vi "主UI.vi"() -> ()   [LabVIEW 2016, in "数据传输系统-03.lvlib" / "自动更新.lvlib" / "TCP文件传输系统.lvlib"]
uses:
  <vilib>/Utility/sysdir.llb/System Directory Type.ctl
panel:
  out "TCP接收全局簇":T1
  out "传输次数":dbl
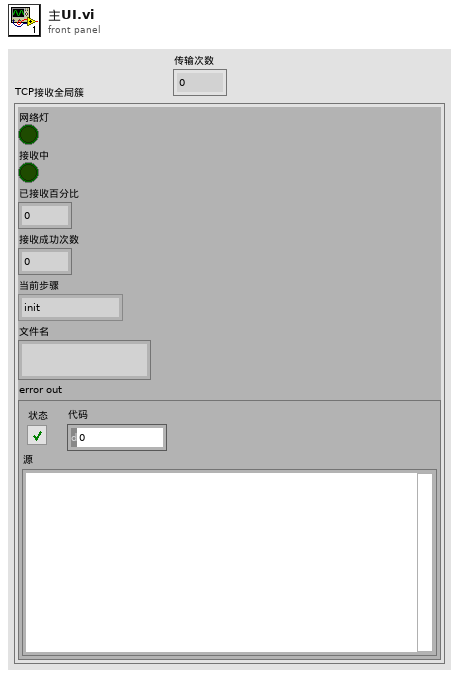
[diagram p1: front panel]
types:
  T1 = cluster{"网络灯":bool, "接收中":bool, "已接收百分比":u8, "接收成功次数":dbl, "当前步骤":enum16{"init", "receivehead", "receivecontent", "receivesuccess", "over"}, "文件名":string, "error out":errorcluster}
  T2 = typedef "System Directory Type.ctl" = i32
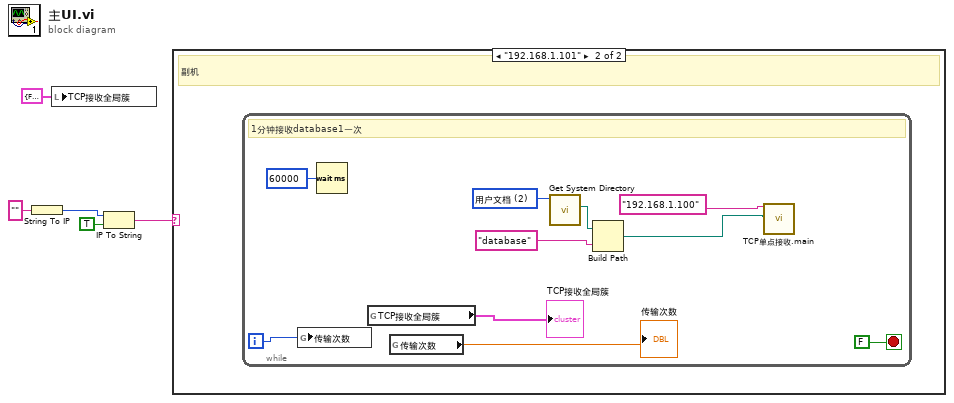
[diagram p0: block diagram]
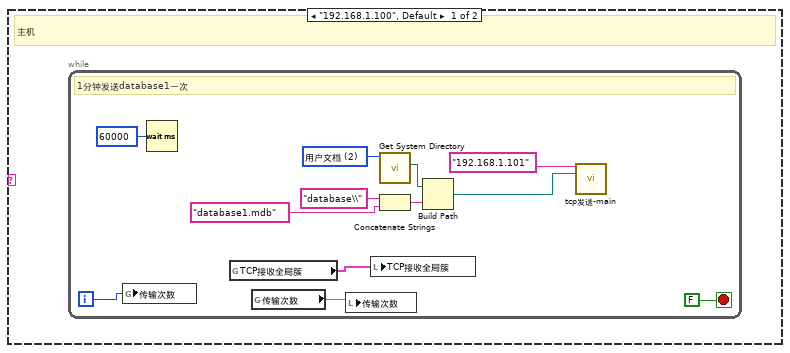
[diagram p2: hidden frame]
diagram:
  n1 = String To IP(1:"" ("名称")) -> (0:w5:u32)
  n2 = local write "TCP接收全局簇"(T1 {"网络灯"=FALSE, "接收中"=FALSE, "已接收百分比"=0, "接收成功次数"=0.0, "当前步骤"=enum."init", "文件名"="", "error out"={"status"=FALSE, "code"=0, "source"=""}} ("TCP接收全局簇")) -> ()
  n3 = IP To String(1:TRUE ("句点符号？(F)"), 2:w5) -> (0:w2:string)
  n4 = case shown="\"192.168.1.101\"" w2 {
    frame "192.168.1.100", Default {
      # "主机"
      n5 = while {
        i -> [w8]
        stop <- FALSE stop-if-true
        w14 = T2 2 items=["用户目录"=0, "用户桌面"=1, "用户文档"=2, "用户应用程序数据"=3, "用户设置"=4, "用户临时目录"=5, "公共文档"=6, "公共应用程序数据"=7, "公共设置"=8, "公共缓存"=13, "系统核心库"=9, "系统安装库"=10, "应用程序文件"=11, "启动盘根目录"=12] ("system directory type")
        # "1分钟发送database1一次"
        n6 = global write "全局变量1.vi" "传输次数"(w8) -> ()
        n7 = Wait (ms)(milliseconds to wait=u32 60000 ("等待时间（毫秒）")) -> ()  [unwired: 1 out]
        n8 = global read "全局变量1.vi" "TCP接收全局簇"() -> (w6:T1)
        n9 = global read "全局变量1.vi" "传输次数"() -> (w7:dbl)
        n10 = local write "传输次数"(w7) -> ()
        n11 = local write "TCP接收全局簇"(w6) -> ()
        n12 = call <vilib>:"Get System Directory.vi"("system directory type"=w14) -> ("system directory"=w13:path)  [unwired: 10 in]
        n13 = Concatenate Strings("database\\" ("condition"), "database1.mdb" ("字符串")) -> (w11:string)
        n14 = Build Path(base path=w13, name or relative path=w11) -> (appended path=w9:path)
        n15 = call "tcp发送-main.vi"("服务器网络地址"="192.168.1.101" ("对方网络地址"), "原文件路径（使用对话框）"=w9) -> ()  [unwired: 12 in, 2 out]
      }
    }
    frame "192.168.1.101" {
      # "副机"
      n16 = while {
        i -> [w21]
        stop <- FALSE stop-if-true
        w25 = T2 2 items=["用户目录"=0, "用户桌面"=1, "用户文档"=2, "用户应用程序数据"=3, "用户设置"=4, "用户临时目录"=5, "公共文档"=6, "公共应用程序数据"=7, "公共设置"=8, "公共缓存"=13, "系统核心库"=9, "系统安装库"=10, "应用程序文件"=11, "启动盘根目录"=12] ("system directory type")
        # "1分钟接收database1一次"
        n17 = global write "全局变量1.vi" "传输次数"(w21) -> ()
        n18 = Wait (ms)(milliseconds to wait=u32 60000 ("等待时间（毫秒）")) -> ()  [unwired: 1 out]
        n19 = global read "全局变量1.vi" "TCP接收全局簇"() -> (→"TCP接收全局簇":T1)
        n20 = global read "全局变量1.vi" "传输次数"() -> (→"传输次数":dbl)
        n21 = call <vilib>:"Get System Directory.vi"("system directory type"=w25) -> ("system directory"=w24:path)  [unwired: 10 in]
        n22 = Build Path(base path=w24, name or relative path="database" ("condition")) -> (appended path=w22:path)
        n23 = call "TCP单点接收.main.vi"("IP地址"="192.168.1.100" ("对方网络地址"), "储存路径"=w22) -> ()  [unwired: 15 in, 3 out]
      }
    }
  }
